vi "ShiftControl.vi"   [LabVIEW 2015]
uses:
  <vilib>/Rock Robotics/WPI/Solenoid/WPI_SolenoidValue.ctl
  Utilities/ShiftGlobals.vi
  <vilib>/Rock Robotics/WPI/Solenoid/WPI_SolenoidSetEnum.vi
types:
  T1 = typedef "WPI_SolenoidDevRef.ctl" = cluster{"DevStatus":errorcluster, "Pneumatics Control Module":u8, "Forward Solenoid Channel":T2, "Reverse Solenoid Channel":T2}
  T2 = typedef "WPI_SolenoidChannel.ctl" = enum8{"Solenoid 0", "Solenoid 1", "Solenoid 2", "Solenoid 3", "Solenoid 4", "Solenoid 5", "Solenoid 6", "Solenoid 7", "Invalid"}
  T3 = typedef "WPI_SolenoidValue.ctl" = enum16{"Off", "On", "Forward", "Reverse"}
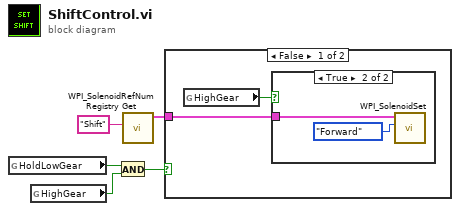
[diagram p0: block diagram]
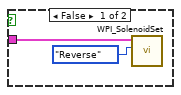
[diagram p2: hidden frame]
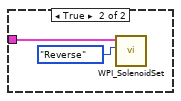
[diagram p3: hidden frame]
diagram:
  n1 = global read "ShiftGlobals.vi" "HoldLowGear"() -> (w3:bool)
  n2 = global read "ShiftGlobals.vi" "HighGear"() -> (w4:bool)
  n3 = And(x=w3, y=w4) -> (x .and. y?=w5:bool)
  n4 = call <vilib>:"WPI_SolenoidRefNum Registry Get.vi"("refnum name"="Shift") -> ("SolenoidDevRef"=w2:T1)  [unwired: 9 in, 1 out]
  n5 = case shown="False" w5 {
    tunnel: w2 -> [w6 w13]
    frame False {
      n6 = global read "ShiftGlobals.vi" "HighGear"() -> (w7:bool)
      n7 = case shown="True" w7 {
        tunnel: w6 -> [w9 w11]
        frame False {
          n8 = call-poly <vilib>:"WPI_SolenoidSet.vi"("Value"=WPI_SolenoidValue."Reverse", "SolenoidDevRef"=w9) -> ()  [unwired: 8 in, 2 out]
        }
        frame True {
          n9 = call-poly <vilib>:"WPI_SolenoidSet.vi"("Value"=WPI_SolenoidValue."Forward", "SolenoidDevRef"=w11) -> ()  [unwired: 8 in, 2 out]
        }
      }
    }
    frame True {
      n10 = call-poly <vilib>:"WPI_SolenoidSet.vi"("Value"=WPI_SolenoidValue."Reverse", "SolenoidDevRef"=w13) -> ()  [unwired: 8 in, 2 out]
    }
  }
